vi "heat_tape_format_data.vi"(9 "t2":dbl, 10 "t1":dbl, 11 "time":timestamp) -> (1 "t_array":dbl[](array[numeric]), 3 "waveform_array":waveform(dbl)[](array[waveform])=[{"t0"=timestamp(0 s since 1904-01-01), "dt"=1.0, "Y"=[]}, {"t0"=timestamp(3732035173.078092 s since 1904-01-01), "dt"=1.0, "Y"=[302.8589782714844], "attributes"=variant("NI_ChannelName"=variant(string "T1"))}])   [LabVIEW 2019]
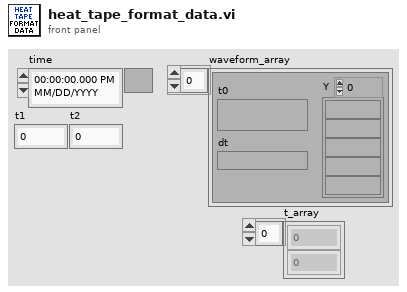
[diagram p1: front panel]
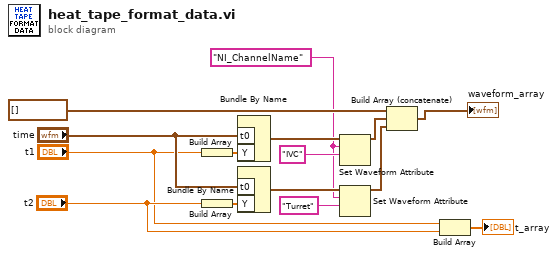
[diagram p0: block diagram]
diagram:
  w4 = "NI_ChannelName" ("name")
  n1 = Build Array("t1") -> (w13:dbl[])
  n2 = Build Array("t2") -> (w10:dbl[])
  n3 = Bundle By Name("t0"="time", "Y"=w13) -> (w12:waveform(dbl))  [unwired: 1 in]
  n4 = Bundle By Name("t0"="time", "Y"=w10) -> (w9:waveform(dbl))  [unwired: 1 in]
  n5 = Set Waveform Attribute(5:"IVC", 6:w4, 7:w12) -> (3:w11:waveform(dbl))  [unwired: 1 in, 2 out]
  n6 = Set Waveform Attribute(5:"Turret", 6:w4, 7:w9) -> (3:w8:waveform(dbl))  [unwired: 1 in, 2 out]
  n7 = Build Array (concatenate)(waveform(dbl)[] [], w11, w8) -> (→"waveform_array":waveform(dbl)[])
  n8 = Build Array("t1", "t2") -> (→"t_array":dbl[])
